vi "CalcularArea.vi"(8 "error in":errorcluster, 11 "object in":refnum<class "Circulo.lvclass">) -> (0 "error out":errorcluster, 2 "Area":dbl, 3 "object out":refnum<class "Circulo.lvclass">)   [LabVIEW 2024, in "Circulo.lvclass"]
uses:
  Circulo.lvclass
  Circulo.lvclass/Circulo.ctl
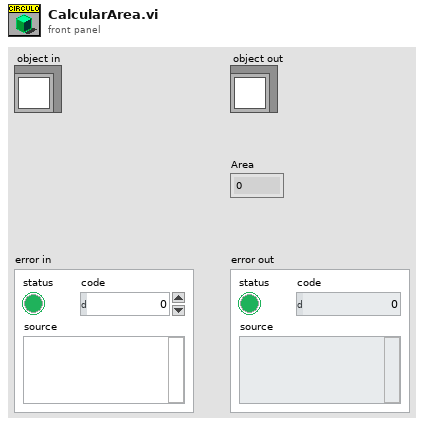
[diagram p1: front panel]
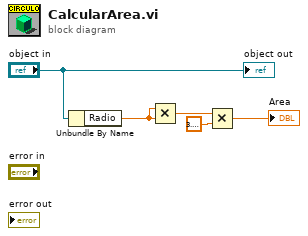
[diagram p0: block diagram]
diagram:
  n1 = Unbundle By Name("object in") -> ("Radio"=w1:dbl)
  n2 = Multiply(x=w1, y=w1) -> (x*y=w3:dbl)
  n3 = Multiply(x=w3, y=3.141592653589793) -> (x*y=→"Area":dbl)
  "object out" <- "object in"
